vi "Get Variable.vi"(8 "error in (no error)":errorcluster, 10 "Name":string, 11 "Sequence in":refnum<class "Sequence.lvclass">) -> (0 "error out":errorcluster, 1 "Value":dbl, 2 "Not Found":bool, 3 "Sequence out":refnum<class "Sequence.lvclass">)   [LabVIEW 2020, in "VolatusSeq.lvlib" / "Sequence.lvclass"]
uses:
  Sequence.lvclass
  Sequence.lvclass/Sequence.ctl
  Variables/Variables.lvclass
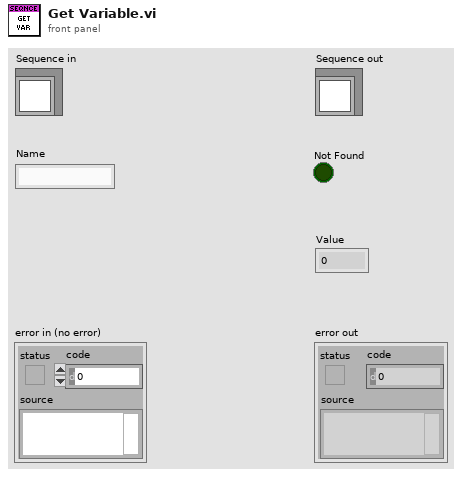
[diagram p1: front panel]
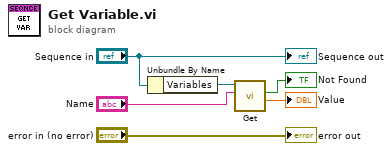
[diagram p0: block diagram]
diagram:
  n1 = Unbundle By Name("Sequence in") -> ("Variables"=w4:refnum<class "Variables.lvclass">)
  n2 = call "Get.vi"("Name"="Name", "Variables in"=w4) -> ("Value"=→"Value":dbl, "Not Found"=→"Not Found":bool)  [unwired: 6 in, 2 out]
  "error out" <- "error in (no error)"
  "Sequence out" <- "Sequence in"
